vi "总氮总磷质控流程.vi"(0 "队列输入TP":refnum<queue>, 5 "总氮量程切换":enum32{"H", "L", "AUTO"}(ring)=enum."AUTO", 7 "总磷量程切换":enum32{"H", "L", "AUTO"}(ring)=enum."AUTO", 9 "总磷":bool, 11 "总氮":bool) -> (4 "布尔":bool, 6 "总磷中断报警":bool, 8 "总氮中断报警":bool)   [LabVIEW 2016, in "质控单元.lvlib"]
panel:
  out "总磷":bool
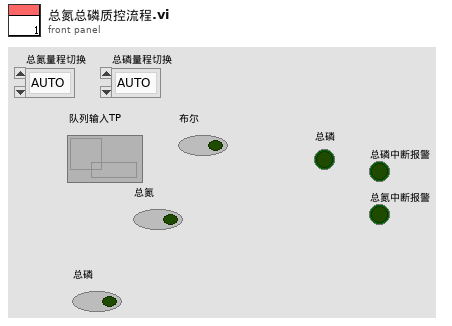
[diagram p1: front panel]
types:
  T1 = enum16{"待机", "启动氨氮水样", "氨氮测量中", "启动氨氮加标", "启动氨氮加标回收", "氨氮加标回收测量中", "启动总氮水样", "总氮测量中", "启动总氮加标", "启动总氮加标回收", "总氮加标回收测量中", "启动总磷水样", "总磷水样测量中", "启动总磷加标", "启动总磷加标回收", "总磷加标回收测量中", "结束"}
  T2 = cluster{"时间标识":timestamp, "设备":string, "日志信息":string}
  T3 = cluster{"站号":u16, "量程切换":enum32{"H", "L", "AUTO"}, "控制命令":enum16{"启动测量", "标样核查", "零点核查", "跨度核查", "空白测试", "平行样测试", "加标回收", "空白校准", "标样校准", "初始化（清洗）", "停止测试", "仪器重启", "校时", "模式设置", "测量间隔设置"}, "模式设置":enum16{"待机", "连续模式", "周期模式", "定点模式", "受控模式", "手动模式"}, "测量间隔":u16}
  T4 = cluster{"系统时间":timestamp, "工作状态":enum16{"空闲", "水样测试", "标样核查", "零点核查", "跨度核查", "空白测试", "平行样测试", "加标回收", "空白校准", "标样校准", "初始化（清洗）"}, "测量模式":enum16{"待机", "连续模式", "周期模式", "定点模式", "受控模式", "手动模式"}, "告警代码":enum16{"无告警", "缺试剂告警", "缺水样告警", "缺蒸馏水告警", "缺标液告警", "仪表漏液告警", "标定异常告警", "超量程告警", "加热异常", "低试剂预警", "超上限告警", "超下限告警", "仪表内部其他异常", "滴定异常告警", "电极异常告警", "量程切换告警", "参数设置告警", "PH电极电位异常", "电导率电极异常", "浊度光度异常", "溶解氧电极异常", "溶解氧光强异常", "温度异常告警", "PH异常告警", "溶解氧异常告警", "电导率异常告警", "浊度异常告警", "叶绿素异常告警", "藻密度异常告警", "蓝绿藻异常告警", "ORP异常告警", "氨氮异常告警", "清洁刷异常告警", "SD卡异常告警", "蓝牙异常告警", "Wifi异常告警", "流程异常告警"}, "故障代码":enum16{"无故障", "电机故障", "温度故障", "通讯故障", "滴定故障"}, "日志代码":u16, "软件版本":u16, "F0":sgl, "F1":sgl, "F2":sgl, "F3":sgl, "T":sgl, "H":sgl, "id":u16, "flowid":u16, "量程":u16, "总磷控温温度1":sgl, "营养盐控温温度2":sgl, "ADC":sgl}
  T5 = enum16{"空闲", "水样测试", "标样核查", "零点核查", "跨度核查", "空白测试", "平行样测试", "加标回收", "空白校准", "标样校准", "初始化（清洗）"}
  T6 = cluster{"因子编码":u32, "单位":u16, "标样参考值":sgl, "水样数据时间":timestamp, "水样实测值":sgl, "水样数据标识":string, "标样数据时间":timestamp, "标样实测值":sgl, "标样数据标识":string, "空白数据时间":timestamp, "空白实测值":sgl, "空白数据标识":string, "零点核查数据时间":timestamp, "零点核查实测值":sgl, "零点核查数据标识":string, "跨度核查数据时间":timestamp, "跨度核查实测值":sgl, "跨度核查数据标识":string, "加标回收数据时间":timestamp, "加标回收实测值":sgl, "加标回收数据标识":string, "平行样数据时间":timestamp, "平行样实测值":sgl, "平行样数据标识":string, "F0":sgl, "F1":sgl, "F2":sgl, "F3":sgl, "F4":sgl, "F5":sgl, "F6":sgl, "F7":sgl, "温度":sgl, "湿度":sgl, "X值":sgl}
  T7 = cluster{"量程":dbl, "检出限":dbl, "加标前水样浓度":dbl, "加标后水样浓度":dbl, "加标水杯定容体积":dbl, "加标母液浓度":dbl, "加标体积":dbl, "加标回收率":dbl}
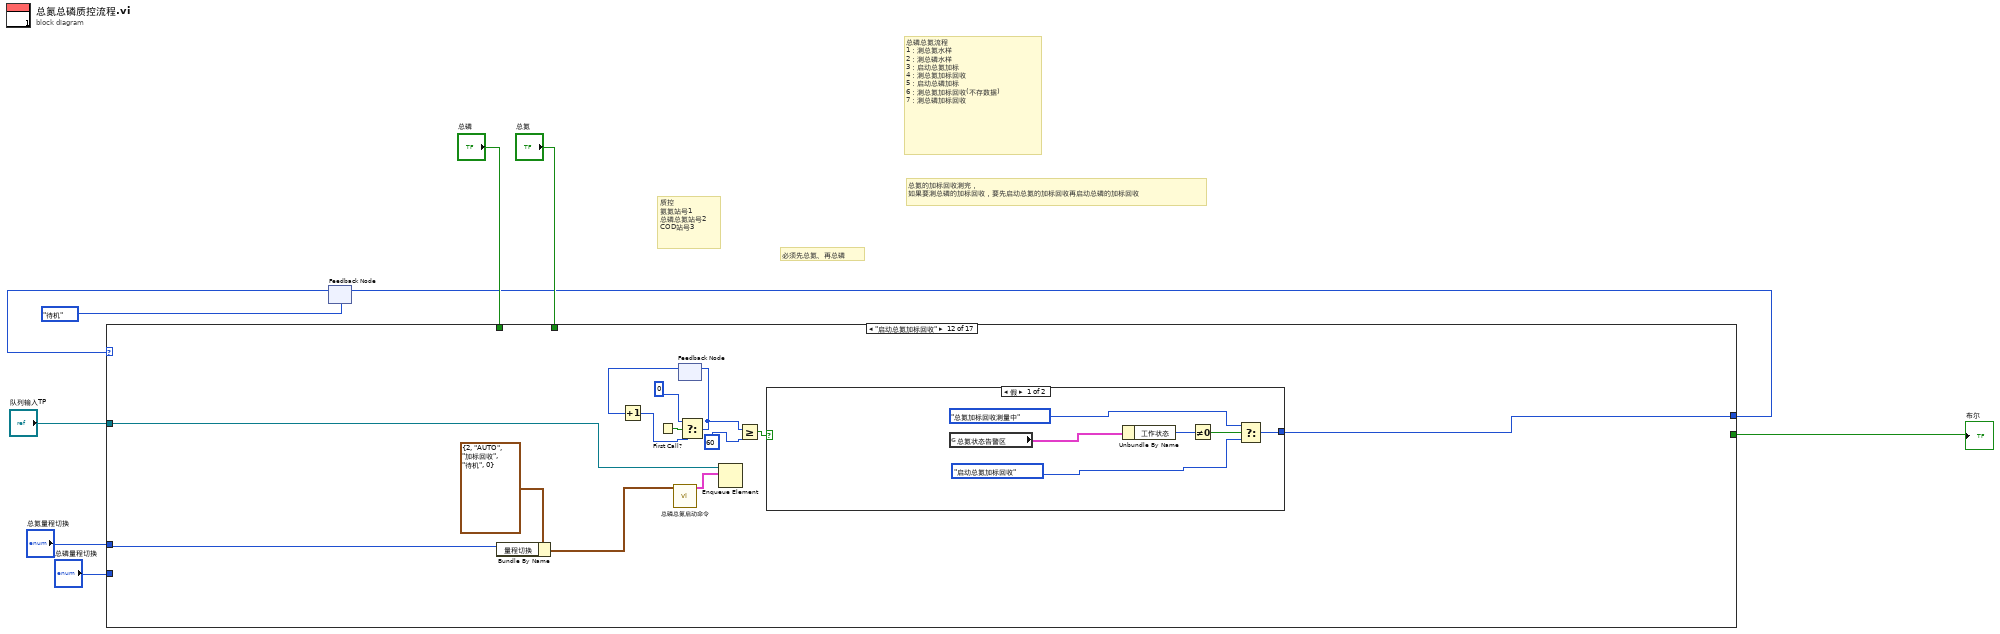
[diagram p0: block diagram]
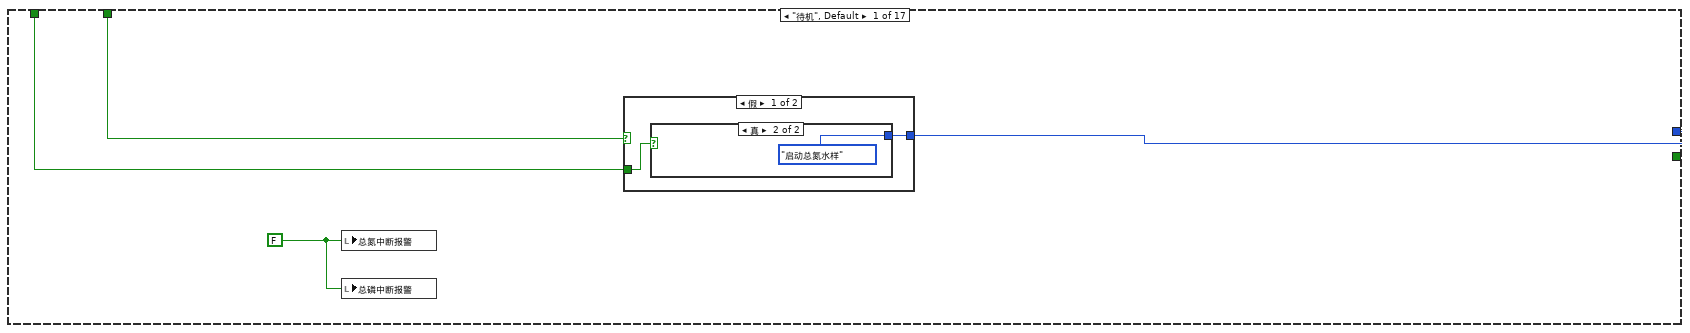
[diagram p2: hidden frame]
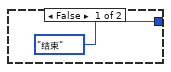
[diagram p3: hidden frame]
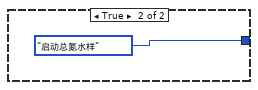
[diagram p4: hidden frame]
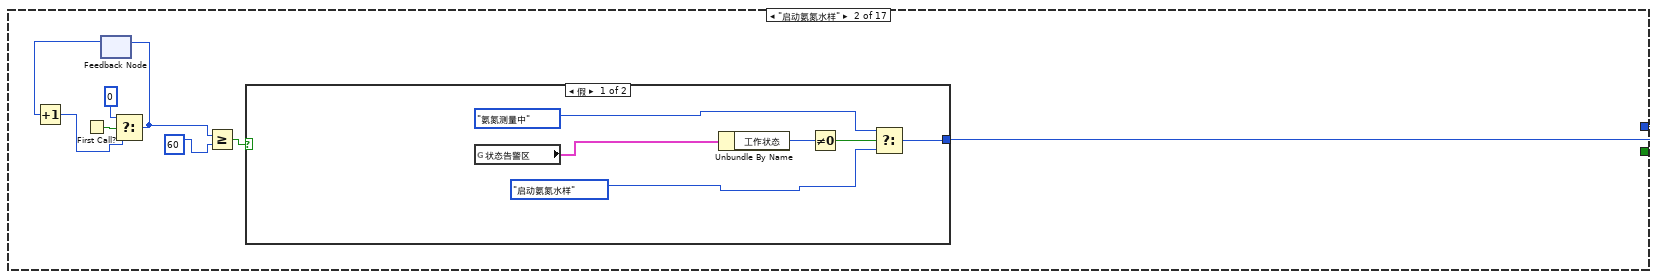
[diagram p5: hidden frame]
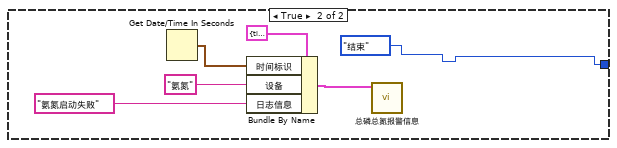
[diagram p6: hidden frame]
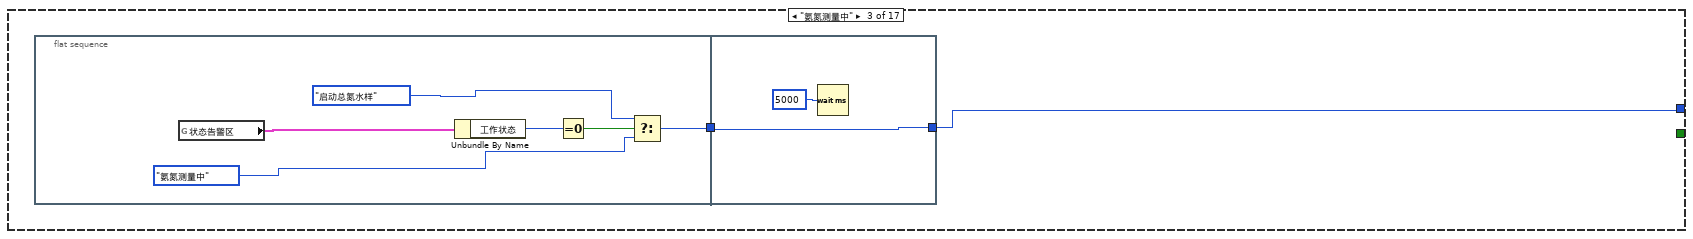
[diagram p7: hidden frame]
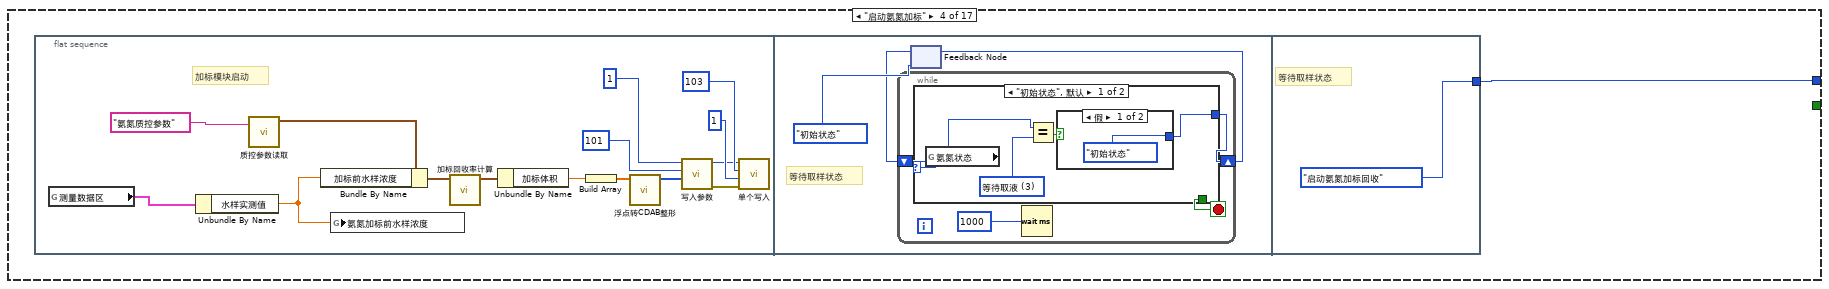
[diagram p8: hidden frame]
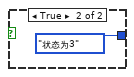
[diagram p9: hidden frame]
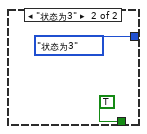
[diagram p10: hidden frame]
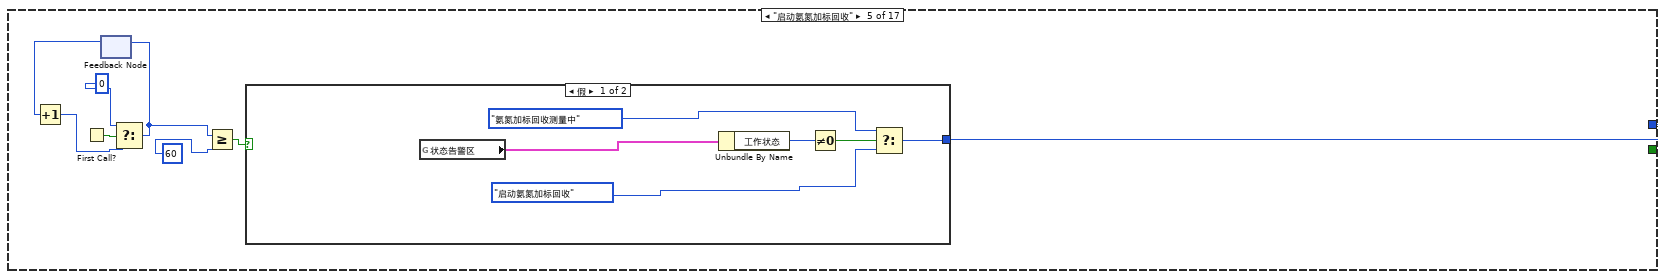
[diagram p11: hidden frame]
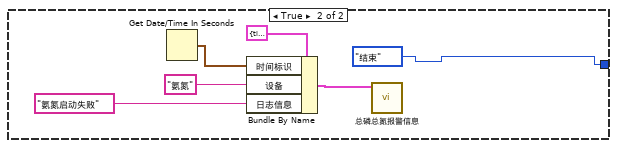
[diagram p12: hidden frame]
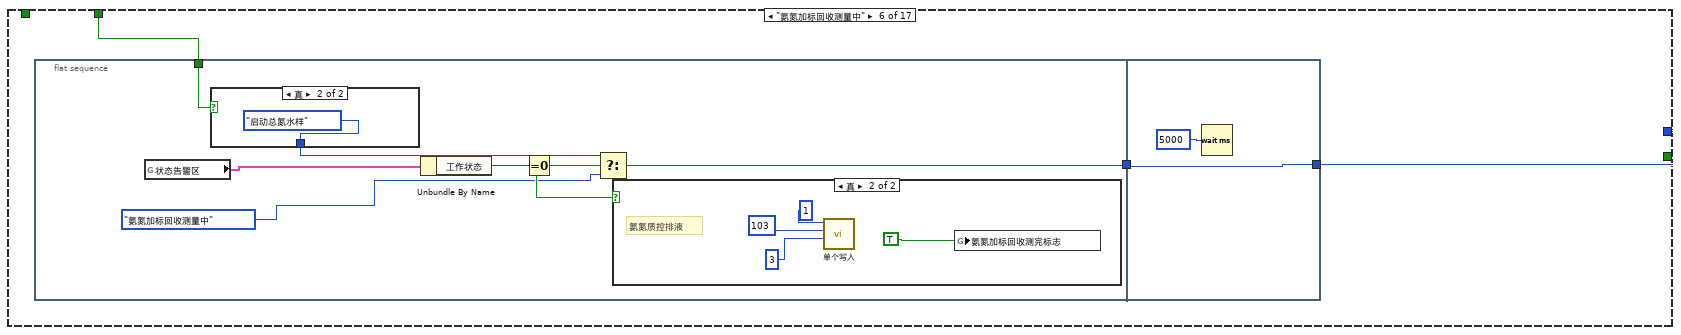
[diagram p13: hidden frame]
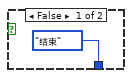
[diagram p14: hidden frame]
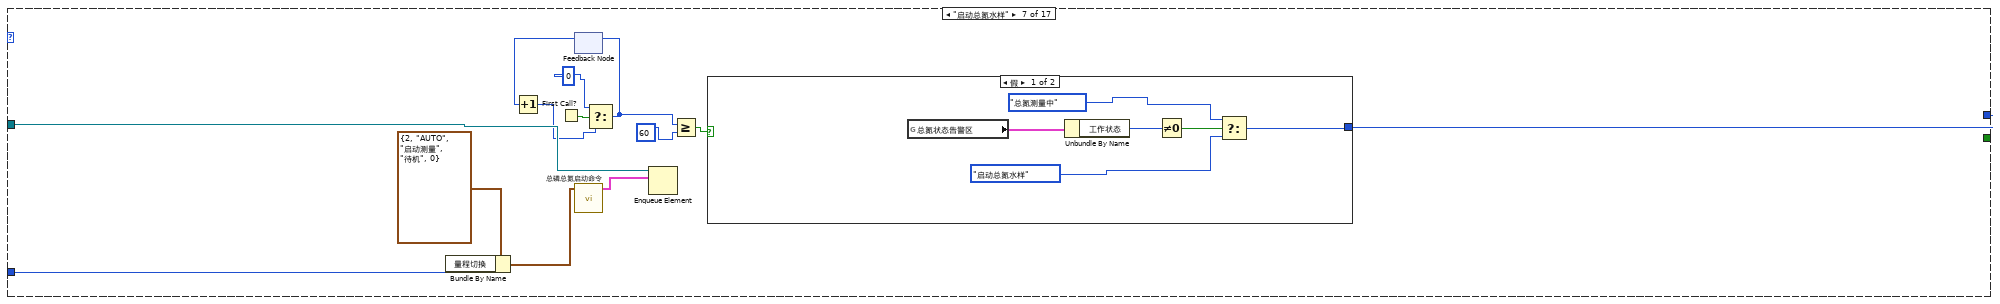
[diagram p16: hidden frame]
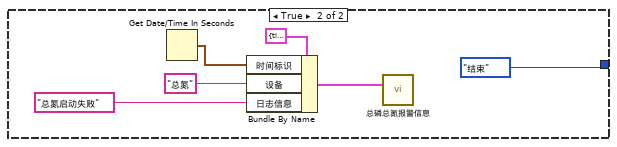
[diagram p17: hidden frame]
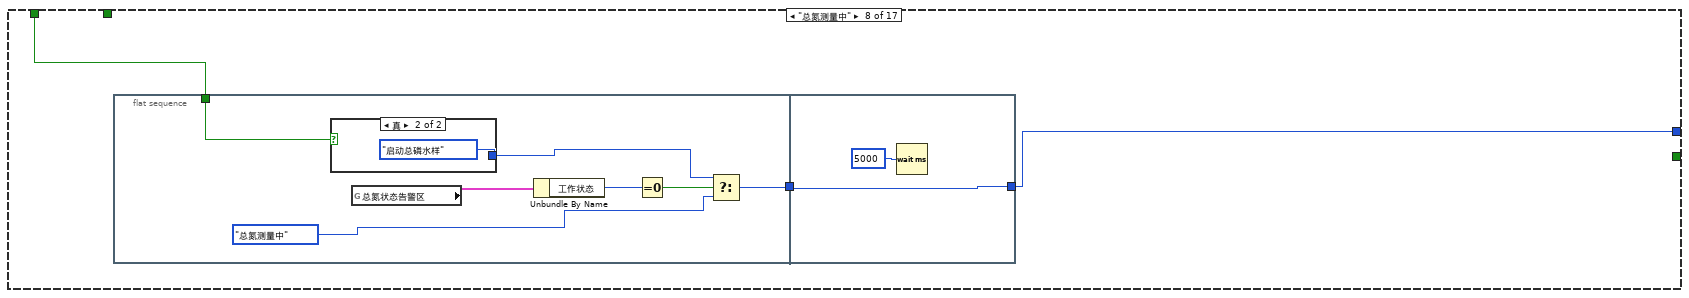
[diagram p18: hidden frame]
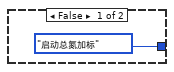
[diagram p19: hidden frame]
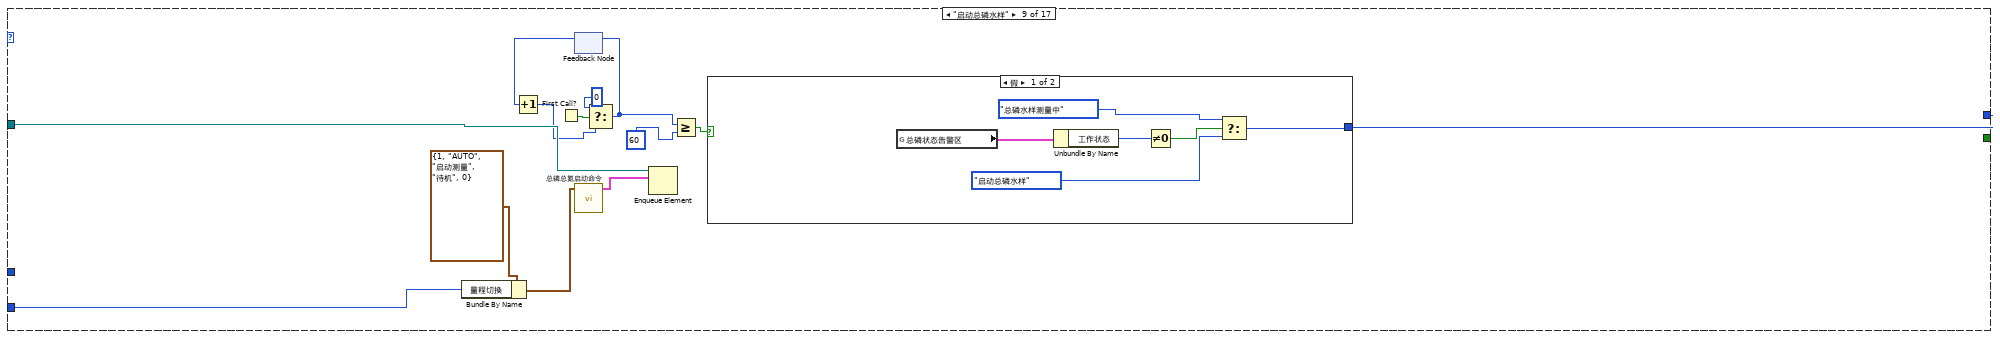
[diagram p20: hidden frame]
diagram:
  # "总磷总氮流程\n1：测总氮水样\n2：测总磷水样\n3：启动总氮加标\n4：测总氮加标回收\n5：启动总磷加标\n6：测总氮加标回收(不存数据)\n7：测总磷加标回收"
  # "总氮的加标回收测完，\n如果要测总磷的加标回收，要先启动总氮的加标回收再启动总磷的加标回收"
  # "质控\n氨氮站号1   \n总磷总氮站号2\nCOD站号3"
  # "必须先总氮、再总磷"
  n1 = feedback #1(T1."待机") -> (w5:T1)
  n2 = case shown="\"启动总氮加标回收\"" w5 {
    tunnel: [w13 w26 w40 w49 w80 w100 w129 w144 w168 w184 w196 w236 w259 w287 w330 w352 T1."结束"] -> w3
    tunnel: "队列输入TP" -> [_ _ _ _ _ _ w130 _ w169 _ _ w238 _ _ w331 _ _]
    tunnel: [_ _ _ _ _ _ _ _ _ _ _ _ _ _ _ _ TRUE] -> w8
    tunnel: "总磷" -> [w12 _ _ _ _ _ _ w143 _ _ _ _ w260 _ _ _ _]
    tunnel: "总氮" -> [w11 _ _ _ _ w101 _ _ _ w182 _ _ w258 _ _ _ _]
    tunnel: "总氮量程切换" -> [_ _ _ _ _ _ w118 _ _ _ _ w233 _ _ _ _ _]
    tunnel: "总磷量程切换" -> [_ _ _ _ _ _ _ _ w157 _ _ _ _ _ w326 _ _]
    frame "待机", Default {
      w10 = FALSE ("总氮中断报警")
      n3 = local write "总氮中断报警"(w10) -> ()
      n4 = local write "总磷中断报警"(w10) -> ()
      n5 = case shown="假" w11 {
        tunnel: w12 -> [w14 _]
        tunnel: [w15 T1."启动总氮水样"] -> w13
        frame False {
          n6 = case shown="真" w14 {
            tunnel: [T1."结束" T1."启动总氮水样"] -> w15
            frame False {
            }
            frame True {
            }
          }
        }
        frame True {
        }
      }
    }
    frame "启动氨氮水样" {
      n7 = First Call?() -> (First Call?: T/F=w24:bool)
      n8 = feedback #2() -> (w23:i32)  [unwired: 1 in]
      n9 = Increment(x=w23) -> (x+1=w22:i32)
      n10 = Select(t=0, s=w24, f=w22) -> (s? t:f=w21:i32)
      n11 = feedback-in #2(w21) -> ()
      n12 = Greater Or Equal?(x=w21, y=60) -> (x >= y?=w19:bool)
      n13 = case shown="假" w19 {
        tunnel: [w30 T1."结束"] -> w26
        frame False {
          n14 = global read "VAR氨氮全局变量.vi" "状态告警区"() -> (w27:T4)
          n15 = Unbundle By Name(w27) -> ("工作状态"=w32:T5)
          n16 = Not Equal To 0?(x=w32) -> (x != 0?=w31:bool)
          n17 = Select(t=T1."氨氮测量中", s=w31, f=T1."启动氨氮水样") -> (s? t:f=w30:T1)
        }
        frame True {
          n18 = Get Date/Time In Seconds() -> (seconds since 1Jan1904=w38:timestamp)
          n19 = Bundle By Name(cluster=T2 {"时间标识"=timestamp(0 s since 1904-01-01), "设备"="", "日志信息"=""} ("data in"), "时间标识"=w38, "设备"="氨氮", "日志信息"="氨氮启动失败") -> (w34:T2)
          n20 = call "总磷总氮报警信息.vi"("data in"=w34) -> ()  [unwired: 10 in, 1 out]
        }
      }
    }
    frame "氨氮测量中" {
      n21 = flat-sequence {
        tunnel: [w45] -> w39
        tunnel: [w48] -> w40
        tunnel: w39 -> [w48]
        frame #0 {
          n22 = global read "VAR氨氮全局变量.vi" "状态告警区"() -> (w41:T4)
          n23 = Unbundle By Name(w41) -> ("工作状态"=w46:T5)
          n24 = Equal To 0?(x=w46) -> (x = 0?=w44:bool)
          n25 = Select(t=T1."启动总氮水样", s=w44, f=T1."氨氮测量中") -> (s? t:f=w45:T1)
        }
        frame #1 {
          n26 = Wait (ms)(milliseconds to wait=u32 5000 ("等待时间（毫秒）")) -> ()  [unwired: 1 out]
        }
      }
    }
    frame "启动氨氮加标" {
      n27 = flat-sequence {
        tunnel: [T1."启动氨氮加标回收"] -> w49
        frame #0 {
          w53 = u16 1 ("value")
          # "加标模块启动"
          n28 = global read "VAR氨氮全局变量.vi" "测量数据区"() -> (w50:T6)
          n29 = Unbundle By Name(w50) -> ("水样实测值"=w51:sgl)
          n30 = call "质控参数读取.vi"("section"="氨氮质控参数") -> ("参数"=w61:T7)  [unwired: 9 in, 1 out]
          n31 = Bundle By Name(cluster=w61, "加标前水样浓度"=w51) -> (w62:T7)
          n32 = global write "水样浓度全局.vi" "氨氮加标前水样浓度"(w51) -> ()
          n33 = call "加标回收率计算.vi"("参数"=w62) -> ("参数 out"=w60:T7)  [unwired: 10 in]
          n34 = Unbundle By Name(w60) -> ("加标体积"=w52:dbl)
          n35 = Build Array(w52) -> (w59:dbl[])
          n36 = call "浮点转CDAB整形.vi"("浮点数"=w59) -> ("CDAB整形输出"=w54:u16[])  [unwired: 10 in]
          n37 = call "写入参数.vi"("values"=w54, "starting address"=u16 101, "Slave ID"=w53) -> ("error out"=w58:errorcluster)  [unwired: 8 in]
          n38 = call "单个写入.vi"("Error in"=w58, "value"=u16 1, "address"=u16 103, "Slave ID"=w53) -> ()  [unwired: 7 in, 1 out]
        }
        frame #1 {
          # "等待取样状态"
          n39 = feedback #3(enum16{"初始状态", "状态为3"}."初始状态") -> (w65:enum16{"初始状态", "状态为3"})
          n40 = while {
            shift-right: [w69] -> w64
            shift-left: w65 -> [w70]
            stop <- w68 stop-if-true
            n41 = case shown="\"初始状态\", 默认" w70 {
              tunnel: [w72 enum16{"初始状态", "状态为3"}."状态为3"] -> w69
              tunnel: [_ TRUE] -> w68
              frame "初始状态", Default {
                w71 = u16 3 items=["待机", "润洗", "进样", "等待取液", "排液"] ("氨氮状态")
                n42 = global read "氨氮加标回收状态全局变量.vi" "氨氮状态"() -> (w74:u16)
                n43 = Equal?(x=w74, y=w71) -> (x = y?=w73:bool)
                n44 = case shown="假" w73 {
                  tunnel: [enum16{"初始状态", "状态为3"}."初始状态" enum16{"初始状态", "状态为3"}."状态为3"] -> w72
                  frame False {
                  }
                  frame True {
                  }
                }
              }
              frame "状态为3" {
              }
            }
            n45 = Wait (ms)(milliseconds to wait=u32 1000 ("等待时间（毫秒）")) -> ()  [unwired: 1 out]
          }
          n46 = feedback-in #3(w64) -> ()
        }
        frame #2 {
          # "等待取样状态"
        }
      }
    }
    frame "启动氨氮加标回收" {
      n47 = First Call?() -> (First Call?: T/F=w86:bool)
      n48 = feedback #4() -> (w85:i32)  [unwired: 1 in]
      n49 = Increment(x=w85) -> (x+1=w84:i32)
      n50 = Select(t=0, s=w86, f=w84) -> (s? t:f=w83:i32)
      n51 = feedback-in #4(w83) -> ()
      n52 = Greater Or Equal?(x=w83, y=60) -> (x >= y?=w81:bool)
      n53 = case shown="假" w81 {
        tunnel: [w91 T1."结束"] -> w80
        frame False {
          n54 = global read "VAR氨氮全局变量.vi" "状态告警区"() -> (w88:T4)
          n55 = Unbundle By Name(w88) -> ("工作状态"=w93:T5)
          n56 = Not Equal To 0?(x=w93) -> (x != 0?=w92:bool)
          n57 = Select(t=T1."氨氮加标回收测量中", s=w92, f=T1."启动氨氮加标回收") -> (s? t:f=w91:T1)
        }
        frame True {
          n58 = Get Date/Time In Seconds() -> (seconds since 1Jan1904=w99:timestamp)
          n59 = Bundle By Name(cluster=T2 {"时间标识"=timestamp(0 s since 1904-01-01), "设备"="", "日志信息"=""} ("data in"), "时间标识"=w99, "设备"="氨氮", "日志信息"="氨氮启动失败") -> (w95:T2)
          n60 = call "总磷总氮报警信息.vi"("data in"=w95) -> ()  [unwired: 10 in, 1 out]
        }
      }
    }
    frame "氨氮加标回收测量中" {
      n61 = flat-sequence {
        tunnel: [w108] -> w102
        tunnel: w101 -> [w105]
        tunnel: [w117] -> w100
        tunnel: w102 -> [w117]
        frame #0 {
          n62 = global read "VAR氨氮全局变量.vi" "状态告警区"() -> (w103:T4)
          n63 = case shown="真" w105 {
            tunnel: [T1."结束" T1."启动总氮水样"] -> w107
            frame False {
            }
            frame True {
            }
          }
          n64 = Unbundle By Name(w103) -> ("工作状态"=w109:T5)
          n65 = Equal To 0?(x=w109) -> (x = 0?=w106:bool)
          n66 = Select(t=w107, s=w106, f=T1."氨氮加标回收测量中") -> (s? t:f=w108:T1)
          n67 = case shown="真" w106 {
            frame False {
            }
            frame True {
              # "氨氮质控排液"
              n68 = call "单个写入.vi"("value"=u16 3, "address"=u16 103, "Slave ID"=u8 1) -> ()  [unwired: 8 in, 1 out]
              n69 = global write "质控测完标志全局 1.vi" "氨氮加标回收测完标志"(TRUE) -> ()
            }
          }
        }
        frame #1 {
          n70 = Wait (ms)(milliseconds to wait=u32 5000 ("等待时间（毫秒）")) -> ()  [unwired: 1 out]
        }
      }
    }
    frame "启动总氮水样" {
      n71 = Bundle By Name(cluster=T3 {"站号"=2, "量程切换"=enum."AUTO", "控制命令"=enum."启动测量", "模式设置"=enum."待机", "测量间隔"=0} ("参数"), "量程切换"=w118) -> (w119:T3)
      n72 = First Call?() -> (First Call?: T/F=w127:bool)
      n73 = feedback #5() -> (w126:i32)  [unwired: 1 in]
      n74 = Increment(x=w126) -> (x+1=w125:i32)
      n75 = call "总磷总氮启动命令.vi"("参数"=w119) -> ("启动命令"=w121:cluster{"命令":string, "data":variant})  [unwired: 10 in]
      n76 = Select(t=0, s=w127, f=w125) -> (s? t:f=w124:i32)
      n77 = feedback-in #5(w124) -> ()
      n78 = Enqueue Element(queue=w130, element=w121) -> ()  [unwired: 2 in, 3 out]
      n79 = Greater Or Equal?(x=w124, y=60) -> (x >= y?=w122:bool)
      n80 = case shown="假" w122 {
        tunnel: [w133 T1."结束"] -> w129
        frame False {
          n81 = global read "VAR总磷总氮全局变量.vi" "总氮状态告警区"() -> (w134:T4)
          n82 = Unbundle By Name(w134) -> ("工作状态"=w135:T5)
          n83 = Not Equal To 0?(x=w135) -> (x != 0?=w136:bool)
          n84 = Select(t=T1."总氮测量中", s=w136, f=T1."启动总氮水样") -> (s? t:f=w133:T1)
        }
        frame True {
          n85 = Get Date/Time In Seconds() -> (seconds since 1Jan1904=w142:timestamp)
          n86 = Bundle By Name(cluster=T2 {"时间标识"=timestamp(0 s since 1904-01-01), "设备"="", "日志信息"=""} ("data in"), "时间标识"=w142, "设备"="总氮", "日志信息"="总氮启动失败") -> (w138:T2)
          n87 = call "总磷总氮报警信息.vi"("data in"=w138) -> ()  [unwired: 10 in, 1 out]
        }
      }
    }
    frame "总氮测量中" {
      n88 = flat-sequence {
        tunnel: [w150] -> w145
        tunnel: w143 -> [w146]
        tunnel: [w156] -> w144
        tunnel: w145 -> [w156]
        frame #0 {
          n89 = case shown="真" w146 {
            tunnel: [T1."启动总氮加标" T1."启动总磷水样"] -> w148
            frame False {
            }
            frame True {
            }
          }
          n90 = global read "VAR总磷总氮全局变量.vi" "总氮状态告警区"() -> (w151:T4)
          n91 = Unbundle By Name(w151) -> ("工作状态"=w152:T5)
          n92 = Equal To 0?(x=w152) -> (x = 0?=w149:bool)
          n93 = Select(t=w148, s=w149, f=T1."总氮测量中") -> (s? t:f=w150:T1)
        }
        frame #1 {
          n94 = Wait (ms)(milliseconds to wait=u32 5000 ("等待时间（毫秒）")) -> ()  [unwired: 1 out]
        }
      }
    }
    frame "启动总磷水样" {
      n95 = Bundle By Name(cluster=T3 {"站号"=1, "量程切换"=enum."AUTO", "控制命令"=enum."启动测量", "模式设置"=enum."待机", "测量间隔"=0} ("参数"), "量程切换"=w157) -> (w158:T3)
      n96 = First Call?() -> (First Call?: T/F=w166:bool)
      n97 = feedback #6() -> (w165:i32)  [unwired: 1 in]
      n98 = Increment(x=w165) -> (x+1=w164:i32)
      n99 = call "总磷总氮启动命令.vi"("参数"=w158) -> ("启动命令"=w160:cluster{"命令":string, "data":variant})  [unwired: 10 in]
      n100 = Select(t=0, s=w166, f=w164) -> (s? t:f=w163:i32)
      n101 = feedback-in #6(w163) -> ()
      n102 = Enqueue Element(queue=w169, element=w160) -> ()  [unwired: 2 in, 3 out]
      n103 = Greater Or Equal?(x=w163, y=60) -> (x >= y?=w161:bool)
      n104 = case shown="假" w161 {
        tunnel: [w172 T1."结束"] -> w168
        frame False {
          n105 = global read "VAR总磷总氮全局变量.vi" "总磷状态告警区"() -> (w173:T4)
          n106 = Unbundle By Name(w173) -> ("工作状态"=w174:T5)
          n107 = Not Equal To 0?(x=w174) -> (x != 0?=w175:bool)
          n108 = Select(t=T1."总磷水样测量中", s=w175, f=T1."启动总磷水样") -> (s? t:f=w172:T1)
        }
        frame True {
          n109 = Get Date/Time In Seconds() -> (seconds since 1Jan1904=w181:timestamp)
          n110 = Bundle By Name(cluster=T2 {"时间标识"=timestamp(0 s since 1904-01-01), "设备"="", "日志信息"=""} ("data in"), "时间标识"=w181, "设备"="总磷", "日志信息"="总磷启动失败") -> (w177:T2)
          n111 = call "总磷总氮报警信息.vi"("data in"=w177) -> ()  [unwired: 10 in, 1 out]
        }
      }
    }
    frame "总磷水样测量中" {
      n112 = flat-sequence {
        tunnel: [w189] -> w183
        tunnel: w182 -> [w186]
        tunnel: [w195] -> w184
        tunnel: w183 -> [w195]
        frame #0 {
          n113 = case shown="真" w186 {
            tunnel: [T1."启动总磷加标" T1."启动总氮加标"] -> w187
            frame False {
            }
            frame True {
            }
          }
          n114 = global read "VAR总磷总氮全局变量.vi" "总磷状态告警区"() -> (w190:T4)
          n115 = Unbundle By Name(w190) -> ("工作状态"=w191:T5)
          n116 = Equal To 0?(x=w191) -> (x = 0?=w188:bool)
          n117 = Select(t=w187, s=w188, f=T1."总磷水样测量中") -> (s? t:f=w189:T1)
        }
        frame #1 {
          n118 = Wait (ms)(milliseconds to wait=u32 7000 ("等待时间（毫秒）")) -> ()  [unwired: 1 out]
        }
      }
    }
    frame "启动总氮加标" {
      n119 = flat-sequence {
        tunnel: [w230] -> w196
        frame #0 {
          w197 = u16 2 ("value")
          # "加标模块启动"
          n120 = global read "VAR总磷总氮全局变量.vi" "总氮测量数据区"() -> (w199:T6)
          n121 = Unbundle By Name(w199) -> ("水样实测值"=w198:sgl)
          n122 = global write "水样浓度全局.vi" "总氮加标前水样浓度"(w198) -> ()
          n123 = call "质控参数读取.vi"("section"="总氮质控参数") -> ("参数"=w201:T7)  [unwired: 9 in, 1 out]
          n124 = Bundle By Name(cluster=w201, "加标前水样浓度"=w198) -> (w210:T7)
          n125 = Wait (ms)(milliseconds to wait=u32 800 ("等待时间（毫秒）")) -> ()  [unwired: 1 out]
          n126 = call "加标回收率计算.vi"("参数"=w210) -> ("参数 out"=w209:T7)  [unwired: 10 in]
          n127 = Unbundle By Name(w209) -> ("加标体积"=w202:dbl)
          n128 = Build Array(w202) -> (w208:dbl[])
          n129 = call "浮点转CDAB整形.vi"("浮点数"=w208) -> ("CDAB整形输出"=w203:u16[])  [unwired: 10 in]
          n130 = call "写入参数.vi"("values"=w203, "starting address"=u16 101, "Slave ID"=w197) -> ("error out"=w207:errorcluster)  [unwired: 8 in]
          n131 = call "单个写入.vi"("Error in"=w207, "value"=u16 1, "address"=u16 103, "Slave ID"=w197) -> ()  [unwired: 7 in, 1 out]
        }
        frame #1 {
          n132 = Wait (ms)(milliseconds to wait=u32 10000 ("等待时间（毫秒）")) -> ()  [unwired: 1 out]
        }
        frame #2 {
          # "等待取样状态"
          n133 = feedback #7(enum16{"初始状态", "状态为3"}."初始状态") -> (w214:enum16{"初始状态", "状态为3"})
          n134 = while {
            shift-right: [w218] -> w213
            shift-left: w214 -> [w219]
            stop <- w217 stop-if-true
            n135 = case shown="\"初始状态\", 默认" w219 {
              tunnel: [w221 enum16{"初始状态", "状态为3"}."状态为3"] -> w218
              tunnel: [_ TRUE] -> w217
              frame "初始状态", Default {
                n136 = global read "氨氮加标回收状态全局变量.vi" "总氮状态"() -> (w220:u16)
                n137 = case shown="3" w220 {
                  tunnel: [enum16{"初始状态", "状态为3"}."状态为3" enum16{"初始状态", "状态为3"}."初始状态" enum16{"初始状态", "状态为3"}."状态为3"] -> w221
                  frame 0 {
                    "总氮中断报警" <- TRUE ("总氮中断报警")
                  }
                  frame 1, Default {
                  }
                  frame 3 {
                    n138 = local write "总氮中断报警"(FALSE ("总氮中断报警")) -> ()
                  }
                }
              }
              frame "状态为3" {
              }
            }
            n139 = Wait (ms)(milliseconds to wait=u32 1000 ("等待时间（毫秒）")) -> ()  [unwired: 1 out]
          }
          n140 = feedback-in #7(w213) -> ()
        }
        frame #3 {
          # "等待取样状态"
          n141 = local read "总氮中断报警"() -> (w229:bool)
          n142 = case shown="假" w229 {
            tunnel: [T1."启动总氮加标回收" T1."结束"] -> w230
            frame False {
            }
            frame True {
            }
          }
        }
      }
    }
    frame "启动总氮加标回收" {
      n143 = Bundle By Name(cluster=T3 {"站号"=2, "量程切换"=enum."AUTO", "控制命令"=enum."加标回收", "模式设置"=enum."待机", "测量间隔"=0} ("参数"), "量程切换"=w233) -> (w234:T3)
      n144 = First Call?() -> (First Call?: T/F=w244:bool)
      n145 = call "总磷总氮启动命令.vi"("参数"=w234) -> ("启动命令"=w237:cluster{"命令":string, "data":variant})  [unwired: 10 in]
      n146 = feedback #8() -> (w243:i32)  [unwired: 1 in]
      n147 = Increment(x=w243) -> (x+1=w242:i32)
      n148 = Select(t=0, s=w244, f=w242) -> (s? t:f=w241:i32)
      n149 = feedback-in #8(w241) -> ()
      n150 = Enqueue Element(queue=w238, element=w237) -> ()  [unwired: 2 in, 3 out]
      n151 = Greater Or Equal?(x=w241, y=60) -> (x >= y?=w239:bool)
      n152 = case shown="假" w239 {
        tunnel: [w248 T1."结束"] -> w236
        frame False {
          n153 = global read "VAR总磷总氮全局变量.vi" "总氮状态告警区"() -> (w251:T4)
          n154 = Unbundle By Name(w251) -> ("工作状态"=w250:T5)
          n155 = Not Equal To 0?(x=w250) -> (x != 0?=w249:bool)
          n156 = Select(t=T1."总氮加标回收测量中", s=w249, f=T1."启动总氮加标回收") -> (s? t:f=w248:T1)
        }
        frame True {
          n157 = Get Date/Time In Seconds() -> (seconds since 1Jan1904=w257:timestamp)
          n158 = Bundle By Name(cluster=T2 {"时间标识"=timestamp(0 s since 1904-01-01), "设备"="", "日志信息"=""} ("data in"), "时间标识"=w257, "设备"="总氮", "日志信息"="总氮启动失败") -> (w253:T2)
          n159 = call "总磷总氮报警信息.vi"("data in"=w253) -> ()  [unwired: 10 in, 1 out]
        }
      }
    }
    frame "总氮加标回收测量中" {
      n160 = flat-sequence {
        tunnel: [w270] -> w261
        tunnel: w260 -> [w267]
        tunnel: w258 -> [w263]
        tunnel: [w286] -> w259
        tunnel: w261 -> [w286]
        frame #0 {
          n161 = case shown="真" w267 {
            tunnel: [T1."结束" w275] -> w269
            tunnel: w263 -> [_ w274]
            frame False {
            }
            frame True {
              n162 = case shown="真" w274 {
                tunnel: [T1."启动总磷加标回收" w278] -> w275
                frame False {
                }
                frame True {
                  n163 = local read "总磷"() -> (w277:bool)
                  n164 = case shown="真" w277 {
                    tunnel: [T1."启动总磷加标" T1."启动总磷加标回收"] -> w278
                    frame False {
                    }
                    frame True {
                    }
                  }
                }
              }
            }
          }
          n165 = global read "VAR总磷总氮全局变量.vi" "总氮状态告警区"() -> (w271:T4)
          n166 = Unbundle By Name(w271) -> ("工作状态"=w272:T5)
          n167 = local read "总磷"() -> (w265:bool)
          n168 = Equal To 0?(x=w272) -> (x = 0?=w268:bool)
          n169 = Not(x=w265) -> (.not. x?=w264:bool)
          n170 = And(x=w268, y=w264) -> (x .and. y?=w262:bool)
          n171 = Select(t=w269, s=w268, f=T1."总氮加标回收测量中") -> (s? t:f=w270:T1)
          n172 = case shown="真" w262 {
            frame False {
            }
            frame True {
              # "总氮质控排液"
              n173 = call "单个写入.vi"("value"=u16 3, "address"=u16 103, "Slave ID"=u8 2) -> ()  [unwired: 8 in, 1 out]
              n174 = global write "质控测完标志全局 1.vi" "总氮加标回收测完标志"(TRUE) -> ()
            }
          }
        }
        frame #1 {
          n175 = Wait (ms)(milliseconds to wait=u32 7000 ("等待时间（毫秒）")) -> ()  [unwired: 1 out]
        }
      }
    }
    frame "启动总磷加标" {
      n176 = flat-sequence {
        tunnel: [w323] -> w287
        frame #0 {
          n177 = Wait (ms)(milliseconds to wait=u32 180000 ("等待时间（毫秒）")) -> ()  [unwired: 1 out]
        }
        frame #1 {
          w294 = u16 2 ("value")
          # "加标模块启动"
          n178 = global read "VAR总磷总氮全局变量.vi" "总磷测量数据区"() -> (w290:T6)
          n179 = Unbundle By Name(w290) -> ("水样实测值"=w289:sgl)
          n180 = call "质控参数读取.vi"("section"="总磷质控参数") -> ("参数"=w292:T7)  [unwired: 9 in, 1 out]
          n181 = Bundle By Name(cluster=w292, "加标前水样浓度"=w289) -> (w302:T7)
          n182 = global write "水样浓度全局.vi" "总磷加标前水样浓度"(w289) -> ()
          n183 = Wait (ms)(milliseconds to wait=u32 800 ("等待时间（毫秒）")) -> ()  [unwired: 1 out]
          n184 = call "加标回收率计算.vi"("参数"=w302) -> ("参数 out"=w301:T7)  [unwired: 10 in]
          n185 = Unbundle By Name(w301) -> ("加标体积"=w293:dbl)
          n186 = Build Array(w293) -> (w300:dbl[])
          n187 = call "浮点转CDAB整形.vi"("浮点数"=w300) -> ("CDAB整形输出"=w295:u16[])  [unwired: 10 in]
          n188 = call "写入参数.vi"("values"=w295, "starting address"=u16 101, "Slave ID"=w294) -> ("error out"=w299:errorcluster)  [unwired: 8 in]
          n189 = call "单个写入.vi"("Error in"=w299, "value"=u16 1, "address"=u16 103, "Slave ID"=w294) -> ()  [unwired: 7 in, 1 out]
        }
        frame #2 {
          n190 = Wait (ms)(milliseconds to wait=u32 10000 ("等待时间（毫秒）")) -> ()  [unwired: 1 out]
        }
        frame #3 {
          # "等待取样状态"
          n191 = feedback #9(enum16{"初始状态", "状态为3"}."初始状态") -> (w306:enum16{"初始状态", "状态为3"})
          n192 = while {
            shift-right: [w310] -> w305
            shift-left: w306 -> [w311]
            stop <- w309 stop-if-true
            n193 = case shown="\"状态为3\"" w311 {
              tunnel: [w313 enum16{"初始状态", "状态为3"}."状态为3"] -> w310
              tunnel: [_ TRUE] -> w309
              frame "初始状态", Default {
                n194 = global read "氨氮加标回收状态全局变量.vi" "总磷状态"() -> (w312:u16)
                n195 = case shown="0" w312 {
                  tunnel: [enum16{"初始状态", "状态为3"}."状态为3" enum16{"初始状态", "状态为3"}."初始状态" enum16{"初始状态", "状态为3"}."状态为3"] -> w313
                  frame 0 {
                    "总磷中断报警" <- TRUE ("总磷中断报警")
                  }
                  frame 1, Default {
                  }
                  frame 3 {
                    n196 = local write "总磷中断报警"(FALSE ("总磷中断报警")) -> ()
                  }
                }
              }
              frame "状态为3" {
                "总磷" <- TRUE
              }
            }
            n197 = Wait (ms)(milliseconds to wait=u32 1000 ("等待时间（毫秒）")) -> ()  [unwired: 1 out]
          }
          n198 = feedback-in #9(w305) -> ()
        }
        frame #4 {
          n199 = local read "总磷中断报警"() -> (w322:bool)
          n200 = case shown="假" w322 {
            tunnel: [T1."启动总氮加标回收" T1."结束"] -> w323
            frame False {
              # "等待取样状态"
            }
            frame True {
            }
          }
        }
      }
    }
    frame "启动总磷加标回收" {
      n201 = Bundle By Name(cluster=T3 {"站号"=1, "量程切换"=enum."AUTO", "控制命令"=enum."加标回收", "模式设置"=enum."待机", "测量间隔"=0} ("参数"), "量程切换"=w326) -> (w327:T3)
      n202 = First Call?() -> (First Call?: T/F=w338:bool)
      n203 = feedback #10() -> (w337:i32)  [unwired: 1 in]
      n204 = Increment(x=w337) -> (x+1=w336:i32)
      n205 = call "总磷总氮启动命令.vi"("参数"=w327) -> ("启动命令"=w332:cluster{"命令":string, "data":variant})  [unwired: 10 in]
      n206 = Select(t=0, s=w338, f=w336) -> (s? t:f=w335:i32)
      n207 = feedback-in #10(w335) -> ()
      n208 = Enqueue Element(queue=w331, element=w332) -> ()  [unwired: 2 in, 3 out]
      n209 = Greater Or Equal?(x=w335, y=60) -> (x >= y?=w333:bool)
      n210 = case shown="假" w333 {
        tunnel: [w342 T1."结束"] -> w330
        frame False {
          n211 = global read "VAR总磷总氮全局变量.vi" "总磷状态告警区"() -> (w343:T4)
          n212 = Unbundle By Name(w343) -> ("工作状态"=w344:T5)
          n213 = Not Equal To 0?(x=w344) -> (x != 0?=w345:bool)
          n214 = Select(t=T1."总磷加标回收测量中", s=w345, f=T1."启动总磷加标回收") -> (s? t:f=w342:T1)
        }
        frame True {
          n215 = Get Date/Time In Seconds() -> (seconds since 1Jan1904=w351:timestamp)
          n216 = Bundle By Name(cluster=T2 {"时间标识"=timestamp(0 s since 1904-01-01), "设备"="", "日志信息"=""} ("data in"), "时间标识"=w351, "设备"="总磷", "日志信息"="总磷启动失败") -> (w347:T2)
          n217 = call "总磷总氮报警信息.vi"("data in"=w347) -> ()  [unwired: 10 in, 1 out]
        }
      }
      n218 = local write "总磷"(FALSE ("总磷")) -> ()
    }
    frame "总磷加标回收测量中" {
      n219 = flat-sequence {
        tunnel: [w357] -> w353
        tunnel: [w365] -> w352
        tunnel: w353 -> [w365]
        frame #0 {
          n220 = global read "VAR总磷总氮全局变量.vi" "总磷状态告警区"() -> (w358:T4)
          n221 = Unbundle By Name(w358) -> ("工作状态"=w359:T5)
          n222 = Equal To 0?(x=w359) -> (x = 0?=w356:bool)
          n223 = Select(t=T1."结束", s=w356, f=T1."总磷加标回收测量中") -> (s? t:f=w357:T1)
          n224 = case shown="真" w356 {
            frame False {
            }
            frame True {
              # "总磷质控排液"
              n225 = global write "质控测完标志全局 1.vi" "总磷加标回收测完标志"(TRUE) -> ()
              n226 = call "单个写入.vi"("value"=u16 3, "address"=u16 103, "Slave ID"=u8 2) -> ()  [unwired: 8 in, 1 out]
            }
          }
        }
        frame #1 {
          n227 = Wait (ms)(milliseconds to wait=u32 5000 ("等待时间（毫秒）")) -> ()  [unwired: 1 out]
        }
      }
    }
    frame "结束" {
      n228 = global write "质控测完标志全局 1.vi" "总氮加标回收测完标志"(FALSE) -> ()
      n229 = global write "质控测完标志全局 1.vi" "总磷加标回收测完标志"(FALSE) -> ()
    }
  }
  "布尔" <- w8
  n230 = feedback-in #1(w3) -> ()
